vi "Globals Demo.vi"() -> ()   [LabVIEW 2015]
panel:
  out "Waveform to FIFO done":bool
  out "Waveform DRAM done":bool
  out "Waveform Exist - Demo":bool
  out "Stop - Demo":bool
  out "Ticks - Demo":bool
  out "Data Index - Demo":i32
  out "Counting Value - Demo":u16
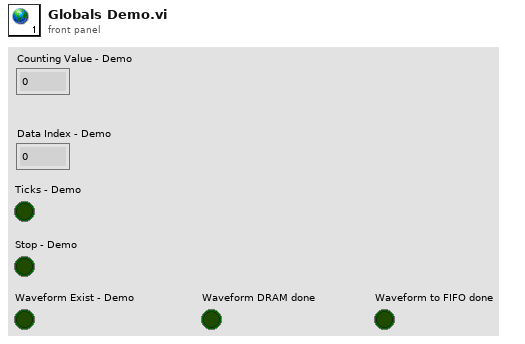
[diagram p1: front panel]
diagram:
